vi "PFI-28000-Channel_Set Type.vi"(8 "error in (no error)":errorcluster, 10 "Type":string, 11 "PFI-28000-Channel in":refnum<class "PFI-28000-Channel.lvclass">) -> (0 "error out":errorcluster, 3 "PFI-28000-Channel out":refnum<class "PFI-28000-Channel.lvclass">)   [LabVIEW 2017, in "PFI-28000-Channel.lvclass"]
uses:
  PFI-28000-Channel.lvclass
  PFI-28000-Channel.lvclass/PFI-28000-Channel.ctl
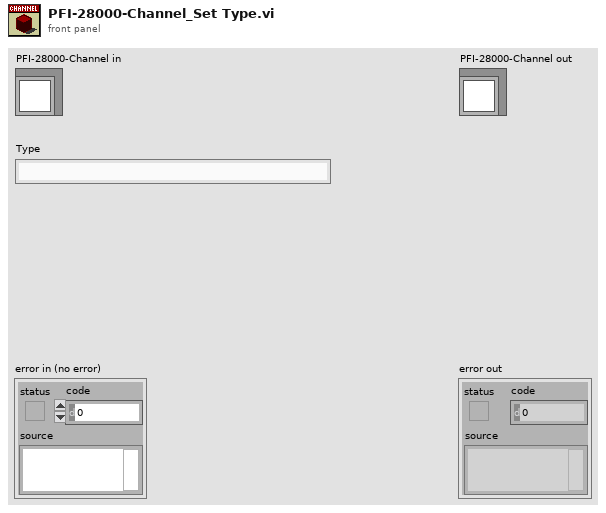
[diagram p1: front panel]
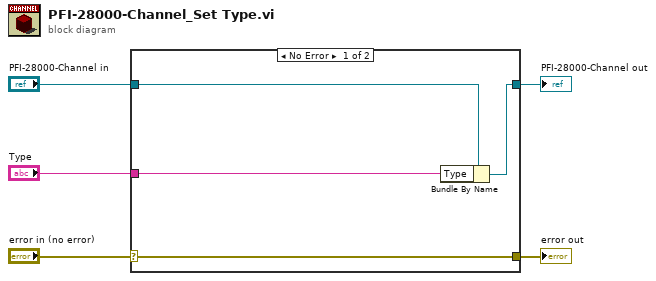
[diagram p0: block diagram]
diagram:
  n1 = case shown="No Error" "error in (no error)" {
    selector: "error in (no error)" -> [w9 w10]
    tunnel: [w9 w10] -> w4
    tunnel: [w7 w11] -> w2
    tunnel: "PFI-28000-Channel in" -> [w8 w11]
    tunnel: "Type" -> [w6 _]
    frame No Error {
      n2 = Bundle By Name(cluster=w8, "Type"=w6) -> (w7:refnum<class "PFI-28000-Channel.lvclass">)
    }
    frame Error {
    }
  }
  "error out" <- w4
  "PFI-28000-Channel out" <- w2
